vi "ImageAnalysis.vi"(8 "error in":errorcluster, 10 "Stop (F)":bool) -> (0 "error out":errorcluster, 1 "Objects bottom cords":T2(array[cluster]), 2 "Walls":T1(array[cluster]))   [LabVIEW 2009, in "Main.lvlib"]
doc: "Main image analysis algorithm. Acquires image from the camera and calculates distances and angles of detected objects."
uses:
  Main.lvlib
  ImageProject/ImageAnalysis.lvlib
  ImageProject/Camera.lvlib
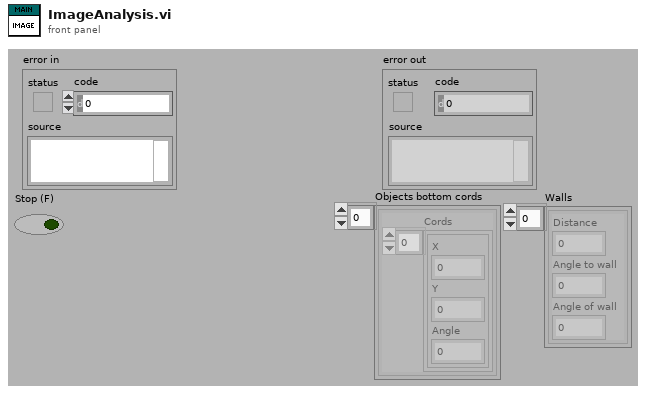
[diagram p1: front panel]
types:
  T1 = cluster{"Distance":dbl, "Angle to wall":dbl, "Angle of wall":dbl}[]
  T2 = cluster{"Cords":cluster{"X":dbl, "Y":dbl, "Angle":dbl}[]}[]
  T3 = typedef "IMAQ Image.ctl" = refnum<image>
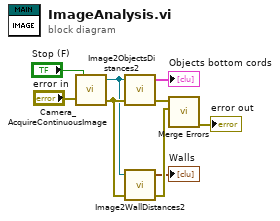
[diagram p0: block diagram]
diagram:
  n1 = call "Camera_AcquireContinuousImage.vi"("Stop (F)"="Stop (F)", "error in"="error in") -> ("Image Out"=w2:T3, "error out"=w8:errorcluster)  [unwired: 1 out]
  n2 = call "Image2ObjectsDistances2.vi"("error in (no error)"=w8, "Image Src"=w2) -> ("error out"=w7:errorcluster, "Objects bottom cords"=→"Objects bottom cords":T2)  [unwired: 2 in]
  n3 = call "Image2WallDistances2.vi"("error in (no error)"=w8, "Image Src"=w2) -> ("error out"=w6:errorcluster, "Walls"=→"Walls":T1)  [unwired: 2 in]
  n4 = call <vilib>:"Merge Errors.vi"("error in 2 (no error)"=w6, "error in 1 (no error)"=w7) -> ("error out"=→"error out":errorcluster)  [unwired: 5 in]
